vi "subGenerateDGMLExternalFolderString.vi"(5 "Apply? (T)":bool=TRUE, 6 "Path in":string="Z:\\OtherFiles", 7 "Expand?":bool, 8 "error in (no error)":errorcluster, 9 "Links in":T1, 10 "Nodes in":T1, 11 "ILabVIEWItem in":refnum<class "ILabVIEWItem.lvclass">) -> (0 "error out":errorcluster, 1 "Links":T1, 2 "Nodes":T1, 3 "ILabVIEWItem out":refnum<class "ILabVIEWItem.lvclass">)   [LabVIEW 2020, in "DefaultExtensions.lvlib" / "CGrapherDGML.lvclass"]
uses:
  CGrapherDGML.lvclass
  obj/Addons/LabVIEWObjectInterfaces.lvlibp/LabVIEWObjectInterfaces/ILabVIEWItem/ILabVIEWItem.lvclass
  obj/Addons/LabVIEWItem.lvlibp/LabVIEWItem/CLabVIEWItem/ConnectionSet.ctl
  ecf4d353-cf80-4459-a486-8bebc84a9ab0.vi
  obj/Addons/LabVIEWItem.lvlibp/LabVIEWItem/CLabVIEWItem/CLabVIEWItem.lvclass
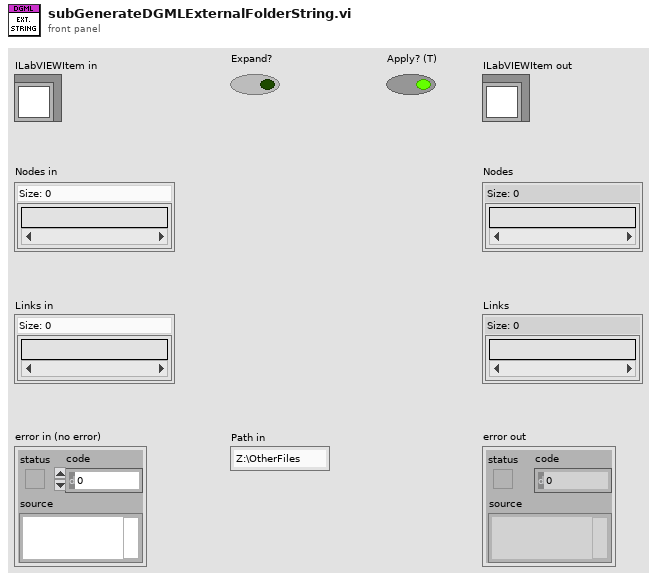
[diagram p1: front panel]
types:
  T1 = typedef "LabVIEWItem.lvlibp/CLabVIEWItem.lvclass/ConnectionSet.ctl" = set{string}
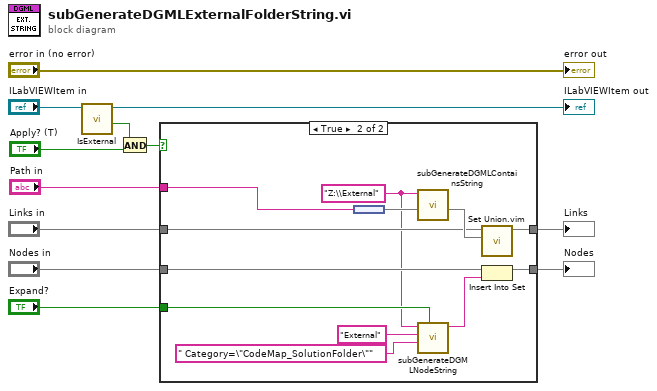
[diagram p0: block diagram]
diagram:
  n1 = call-dynamic "IsExternal.vi"("ILabVIEWItem in"="ILabVIEWItem in") -> ("Is external?"=w3:bool, "ILabVIEWItem out"=→"ILabVIEWItem out":refnum<class "ILabVIEWItem.lvclass">)  [unwired: 8 in, 1 out]
  n2 = And(x=w3, y="Apply? (T)") -> (x .and. y?=w1:bool)
  n3 = case shown="True" w1 {
    tunnel: [w14 w21] -> w10
    tunnel: "Links in" -> [w14 w20]
    tunnel: "Nodes in" -> [w13 w19]
    tunnel: [w13 w18] -> w7
    tunnel: "Expand?" -> [_ w17]
    tunnel: "Path in" -> [_ w16]
    frame False {
    }
    frame True {
      w15 = "Z:\\External" ("format string")
      n4 = node(w16) -> (w26:set{string})
      n5 = call "subGenerateDGMLContainsString.vi"("Contained"=w26, "Source"=w15) -> ("Links"=w25:T1)  [unwired: 9 in]
      n6 = call "subGenerateDGMLNodeString.vi"("Expand?"=w17, "Code schema"=" Category=\"CodeMap_SolutionFolder\"" ("format string"), "Label"="External" ("format string"), "Id"=w15) -> ("Node string"=w23:string)  [unwired: 7 in]
      n7 = call "Set Union.vim"("set 2"=w25, "set 1"=w20) -> ("union"=w21:T1)  [unwired: 9 in]
      n8 = Insert Into Set(10:w23, 11:w19) -> (3:w18:T1)  [unwired: 1 out]
    }
  }
  "Links" <- w10
  "Nodes" <- w7
  "error out" <- "error in (no error)"
